vi "GetYawPitchRollCompass.vi"(0 "Nav6DevRef":T1, 5 "error in (no error)":errorcluster) -> (12 "Yaw (Raw)":dbl, 14 "Nav6DevRef Out":T1, 15 "Yaw":dbl, 16 "Pitch":dbl, 17 "Roll":dbl, 18 "Compass Heading":dbl, 19 "error out":errorcluster)   [LabVIEW 2014, in "Nav6.lvlib"]
doc: "Returns the Yaw, Pitch, Roll, and Compass Heading from the Nav6 in YPR mode. \n\nSee https://code.google.com/p/nav6/wiki/Orientation for a picture of the orientation of the axes."
uses:
  Nav6.lvlib
  Nav6DevRef.ctl
  <vilib>/Rock Robotics/WPI/SerialPort/WPI_SerialPortRef.ctl
  Nav6Mode.ctl
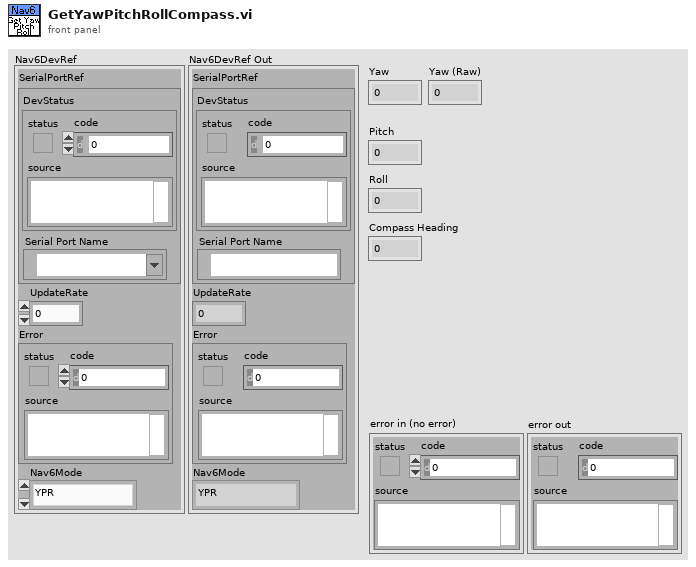
[diagram p1: front panel]
types:
  T1 = typedef "Nav6.lvlib/Nav6DevRef.ctl" = cluster{"SerialPortRef":T2, "UpdateRate":u8, "Error":errorcluster, "Nav6Mode":T3}
  T2 = typedef "WPI_SerialPortRef.ctl" = cluster{"DevStatus":errorcluster, "Serial Port Name":refnum<visa-resource-name>}
  T3 = typedef "Nav6.lvlib/Nav6Mode.ctl" = enum16{"YPR", "Gyro", "Quaternion"}
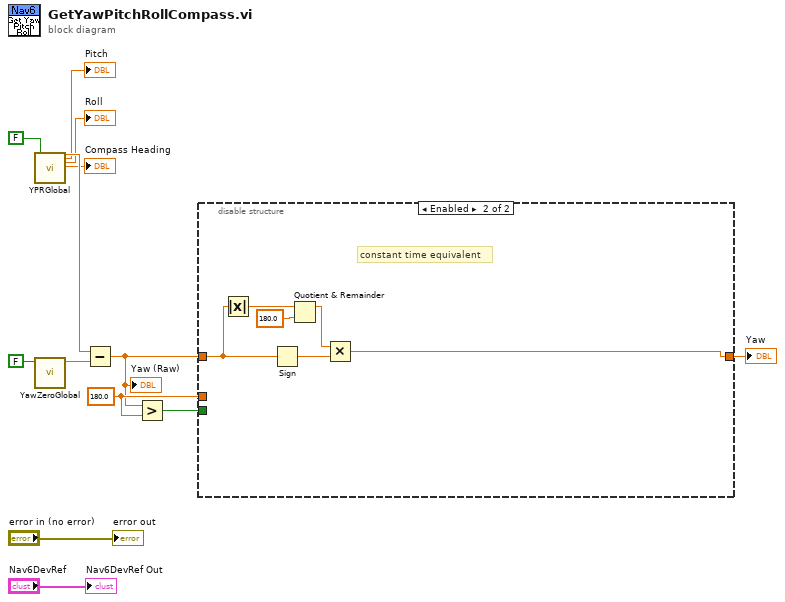
[diagram p0: block diagram]
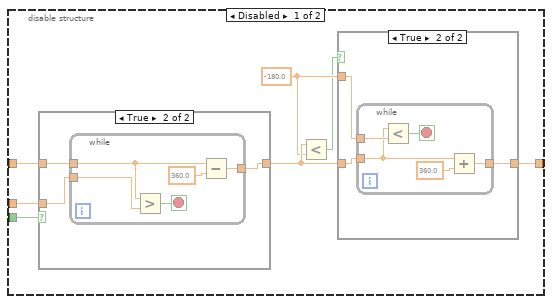
[diagram p2: hidden frame]
diagram:
  w10 = 180.0 ("y")
  n1 = call "YPRGlobal.vi"("Update"=FALSE) -> ("Yaw Out"=w12:dbl, "Pitch Out"=→"Pitch":dbl, "Roll Out"=→"Roll":dbl, "Compass Heading Out"=→"Compass Heading":dbl)  [unwired: 20 in, 3 out]
  n2 = call "YawZeroGlobal.vi"("Update"=FALSE) -> ("YawZero"=w11:dbl)  [unwired: 10 in]
  n3 = Subtract(x=w12, y=w11) -> (x-y=w1:dbl)
  "Yaw (Raw)" <- w1
  n4 = Greater?(x=w1, y=w10) -> (0:w7:bool)
  n5 = disable-structure shown="Enabled" {
    disable-tunnel: w10 -> [w20 _]
    disable-tunnel: [w19 w39] -> w9
    disable-tunnel: w7 -> [w18 _]
    disable-tunnel: w1 -> [w14 w40]
    frame Disabled {
      w16 = -180.0 ("y")
      n6 = case shown="True" w18 {
        tunnel: w14 -> [w30 w33]
        tunnel: [w30 w31] -> w17
        tunnel: w20 -> [_ w32]
        frame False {
        }
        frame True {
          n7 = while {
            tunnel: w33 -> [w35]
            tunnel: w32 -> [w37]
            tunnel: [w36] -> w31
            stop <- w38 stop-if-true
            n8 = Greater?(x=w35, y=w37) -> (0:w38:bool)
            n9 = Subtract(x=w35, y=360.0) -> (x-y=w36:dbl)
          }
        }
      }
      n10 = Less?(x=w17, y=w16) -> (x < y?=w15:bool)
      n11 = case shown="True" w15 {
        tunnel: w17 -> [w21 w24]
        tunnel: [w21 w22] -> w19
        tunnel: w16 -> [_ w23]
        frame False {
        }
        frame True {
          n12 = while {
            tunnel: w24 -> [w26]
            tunnel: w23 -> [w28]
            tunnel: [w27] -> w22
            stop <- w29 stop-if-true
            n13 = Less?(x=w26, y=w28) -> (x < y?=w29:bool)
            n14 = Add(x=w26, y=360.0) -> (x+y=w27:dbl)
          }
        }
      }
    }
    frame Enabled {
      # "constant time equivalent"
      n15 = Absolute Value(x=w40) -> (abs(x)=w42:dbl)
      n16 = Sign(1:w40) -> (0:w44:dbl)
      n17 = Quotient & Remainder(x=w42, y=180.0) -> (x-y*floor(x/y)=w43:dbl)  [unwired: 1 out]
      n18 = Multiply(x=w43, y=w44) -> (x*y=w39:dbl)
    }
  }
  "Yaw" <- w9
  "Nav6DevRef Out" <- "Nav6DevRef"
  "error out" <- "error in (no error)"
